vi "Read Content.vi"(8 "Error In":errorcluster, 11 "EscapedTag In":refnum<class "EscapedTag.lvclass">) -> (0 "Error Out":errorcluster, 2 "Content":string, 3 "EscapedTag Out":refnum<class "EscapedTag.lvclass">)   [LabVIEW 2018, in "Toolkit.lvlib" / "Nodes.lvlib" / "EscapedTag.lvclass"]
uses:
  EscapedTag.lvclass
  NonTerminal/NonTerminal.lvclass
  EscapedTag.lvclass/EscapedTag.ctl
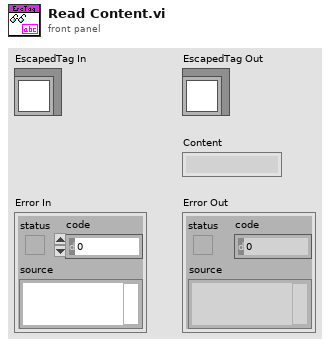
[diagram p1: front panel]
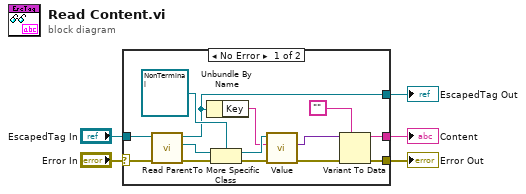
[diagram p0: block diagram]
diagram:
  n1 = case shown="No Error" "Error In" {
    selector: "Error In" -> [w18 w20]
    tunnel: "EscapedTag In" -> [w19 w21]
    tunnel: [w12 w21] -> w3
    tunnel: [w9 w20] -> w2
    tunnel: [w6 _] -> w1
    frame No Error {
      n2 = call-dynamic "Read Parent.vi"("Error In"=w18, "Terminal In"=w19) -> ("Error Out"=w17:errorcluster, "Parent"=w16:refnum<class "Abstract.lvclass">, "Terminal Out"=w12:refnum<class "EscapedTag.lvclass">)  [unwired: 7 in]
      n3 = Unbundle By Name(w12) -> ("Key"=w11:string)
      n4 = To More Specific Class(target class=refnum<class "NonTerminal.lvclass"> refnum ("Toolkit.lvlib:Nodes.lvlib:NonTerminal.lvclass"), reference=w16, error in=w17) -> (specific class reference=w14:refnum<class "NonTerminal.lvclass">, error out=w13:errorcluster)
      n5 = call-dynamic "Value.vi"("Error In"=w13, "Key"=w11, "Non-Terminal In"=w14) -> ("Error Out"=w10:errorcluster, "Value"=w8:variant)  [unwired: 6 in, 1 out]
      n6 = Variant To Data(error in=w10, type="", Variant=w8) -> (data=w6:string, error out=w9:errorcluster)
    }
    frame Error {
    }
  }
  "Error Out" <- w2
  "EscapedTag Out" <- w3
  "Content" <- w1
